vi "LogUserEvent.vi"(8 "error in":errorcluster caption="错误输入（无错误）", 9 "StrIn":string, 11 "Event":string) -> (0 "error out":errorcluster caption="错误输出")   [LabVIEW 2013]
uses:
  Ctl/Logctl.ctl
  Global.vi
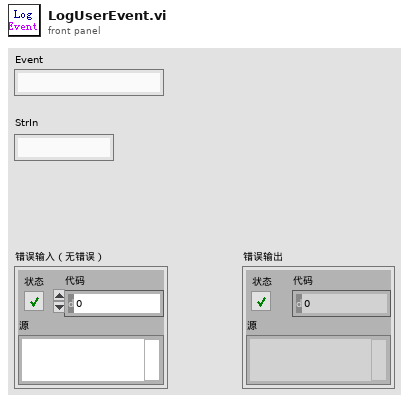
[diagram p1: front panel]
types:
  T1 = typedef "Logctl.ctl" = cluster{"Event":string, "Value":variant}
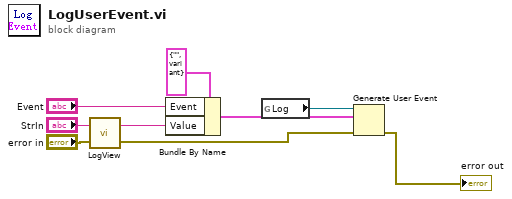
[diagram p0: block diagram]
diagram:
  n1 = call "LogView.vi"("error in"="error in", "StrIn"="StrIn") -> ("error out"=w1:errorcluster, "StrOut"=w3:string)
  n2 = Bundle By Name(cluster=T1 {"Event"="", "Value"=variant} ("Log"), "Event"="Event", "Value"=w3) -> (w7:T1)
  n3 = global read "Global.vi" "Log"() -> (w8:refnum<user-event>)
  n4 = Generate User Event(user event=w8, event data cluster=w7, error in=w1) -> (error out=→"error out":errorcluster)  [unwired: 1 in, 1 out]
